vi "ADIS16470 Loop Custom.vi"(8 "error in":errorcluster) -> ()   [LabVIEW 2019]
uses:
  Typedef/ADIS16470 Hardware Configuration.ctl
  <vilib>/Rock Robotics/WPI/SPI/WPI_SPIMode.ctl
  <vilib>/Rock Robotics/SystemInterfaces/DIO/FPGA_DIOChannel.ctl
  <vilib>/Rock Robotics/SystemInterfaces/spilib/spi_bus.ctl
  Typedef/ADIS16470 Process.ctl
  Typedef/ADIS16470 Device Reference.ctl
  Typedef/ADIS16470 Data.ctl
  Typedef/ADIS16470 Status.ctl
  Typedef/ADIS16470 Command Type.ctl
  <vilib>/Rock Robotics/WPI/SPI/WPI_SPIDevRef.ctl
  <vilib>/Rock Robotics/WPI/Interrupt/WPI_InterruptRef.ctl
  <vilib>/Rock Robotics/SystemInterfaces/Interrupt/FPGA_InterruptIndex.ctl
  <vilib>/Rock Robotics/WPI/Encoder/WPI_EncoderDevRef.ctl
  <vilib>/Rock Robotics/SystemInterfaces/Encoder/FPGA_EncoderIdx.ctl
  <vilib>/Rock Robotics/SystemInterfaces/Counter/FPGA_CounterCtrSystemIndex.ctl
  <vilib>/Rock Robotics/WPI/Encoder/WPI_EncoderType.ctl
  <vilib>/Rock Robotics/SystemInterfaces/NetworkCommunication/NetComm_UsageReport_ResourceType.ctl
  Typedef/ADIS16470 Register.ctl
  <vilib>/Rock Robotics/WPI/Counter/WPI_CounterDigitalInputToDigitalSource.vi
  <vilib>/Rock Robotics/SystemInterfaces/CounterEncoderSourceConvertion/FPGA_CounterEncoderSourceConvertionLVSourceTypeToFPGAType.vi
  <vilib>/Rock Robotics/WPI/Interrupt/WPI_InterruptCache.vi
  <vilib>/Rock Robotics/SystemInterfaces/Interrupt/FPGA_InterruptWriteConfiguration.vi
  <vilib>/Rock Robotics/SystemInterfaces/Interrupt/FPGA_WaitOnInterrupt.vi
  <vilib>/Rock Robotics/WPI/Utilities/WPI_UtilitiesTimebaseConstants.vi
  <vilib>/Rock Robotics/SystemInterfaces/Interrupt/FPGA_InterruptReadTimestamp.vi
panel:
  in  "Sychronous Process VI":T1
  in  "Hardware Config":T2={"SPI Clock Rate (Hz)"=2000000.0, "IMU SPI Mode (3)"=enum."Mode 3 (Clk Idle High,Sample on Trailing)", "IMU Reset Pin"=enum."SPI Port CS2", "IMU SPI Bus"=enum."SPI On-Board, CS0", "IMU Data Ready Pin"=enum."SPI Port CS1"}
  out "Waveform Chart":dbl(graph)
  out "Offset Bias":i16[](array[numeric])
  out "xAngle":dbl
  out "yAngle":dbl
  out "Data":dbl[](array[numeric])
  out "Counter":u16
  # "x"
  # "y"
  # "z"
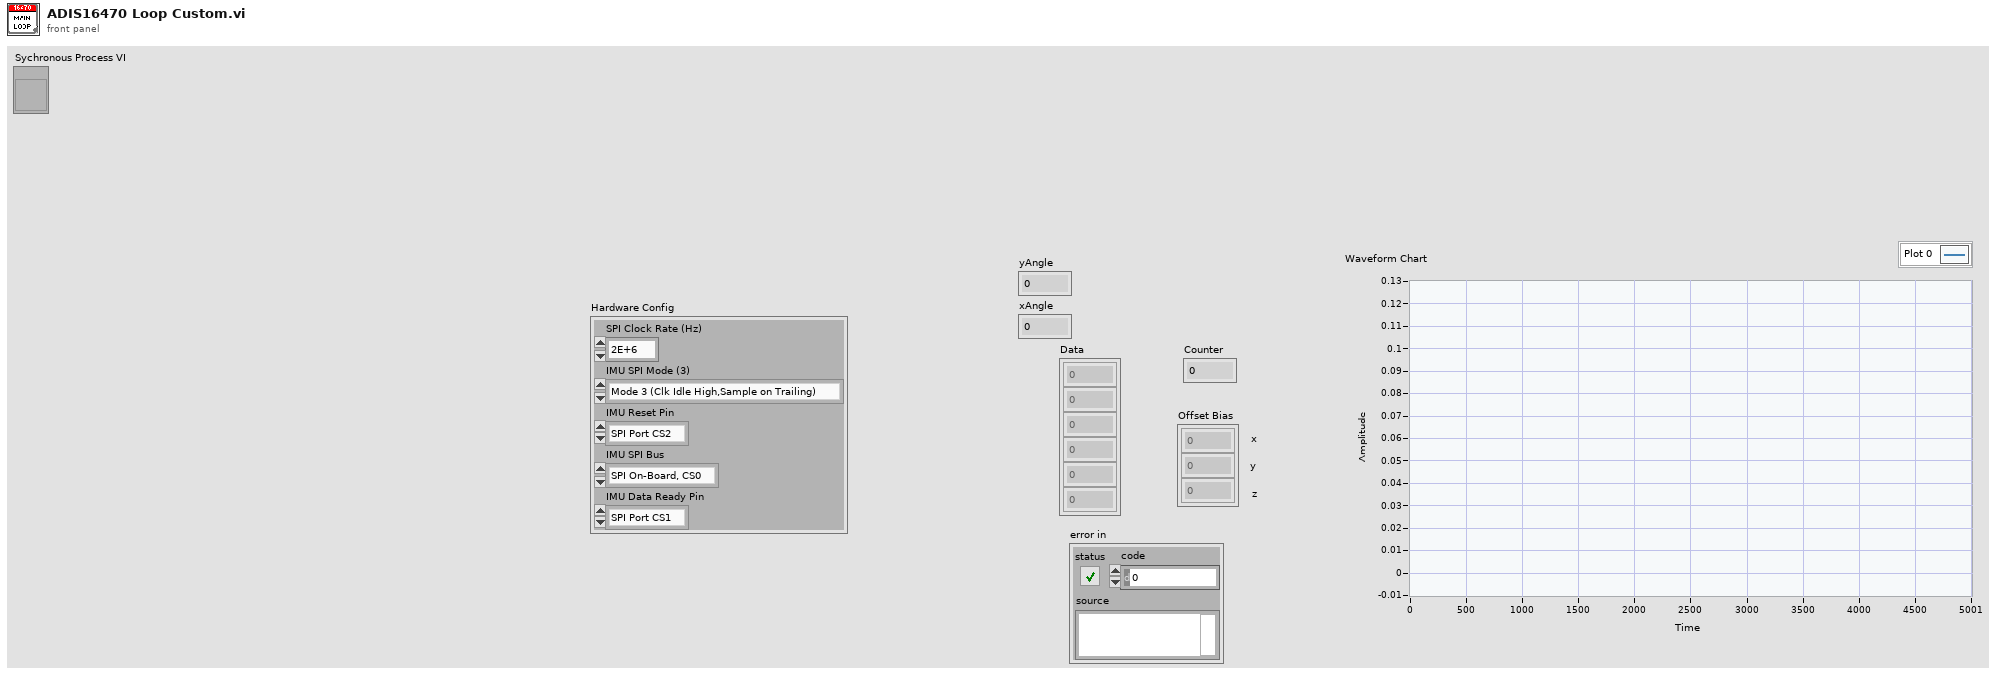
[diagram p1: front panel]
types:
  T1 = typedef "ADIS16470 Process.ctl" = refnum<vi>
  T2 = typedef "ADIS16470 Hardware Configuration.ctl" = cluster{"SPI Clock Rate (Hz)":dbl, "IMU SPI Mode (3)":T3, "IMU Reset Pin":T4, "IMU SPI Bus":T5, "IMU Data Ready Pin":T4}
  T3 = typedef "WPI_SPIMode.ctl" = enum16{"Mode 0 (Clk Idle Low,Sample on Leading)", "Mode 1 (Clk Idle Low,Sample on Trailing)", "Mode 2 (Clk Idle High,Sample on Leading)", "Mode 3 (Clk Idle High,Sample on Trailing)"}
  T4 = typedef "FPGA_DIOChannel.ctl" = enum8{"DIO 0", "DIO 1", "DIO 2", "DIO 3", "DIO 4", "DIO 5", "DIO 6", "DIO 7", "DIO 8", "DIO 9", "DIO MXP 0", "DIO MXP 1", "DIO MXP 2", "DIO MXP 3", "DIO MXP 4", "DIO MXP 5", "DIO MXP 6", "DIO MXP 7", "DIO MXP 8", "DIO MXP 9", "DIO MXP 10", "DIO MXP 11", "DIO MXP 12", "DIO MXP 13", "DIO MXP 14", "DIO MXP 15", "SPI Port CS1", "SPI Port CS2", "SPI Port CS3", "SPI Port MISO", "SPI Port MOSI", "Invalid"}
  T5 = typedef "spi_bus.ctl" = enum16{"SPI On-Board, CS0", "SPI On-Board, CS1", "SPI On-Board, CS2", "SPI On-Board, CS3", "SPI MXP", "Invalid"}
  T6 = typedef "NetComm_UsageReport_ResourceType.ctl" = enum8{"Controller", "Module", "Language", "CANPlugin", "Accelerometer", "ADXL345", "AnalogChannel", "AnalogTrigger", "AnalogTriggerOutput", "CANJaguar", "Compressor", "Counter", "Dashboard", "DigitalInput", "DigitalOutput", "DriverStationCIO", "DriverStationEIO", "DriverStationLCD", "Encoder", "GearTooth", "Gyro", "I2C", "Framework", "Jaguar", "Joystick", "Kinect", "KinectStick", "PIDController", "Preferences", "PWM", "Relay", "RobotDrive", "SerialPort", "Servo", "Solenoid", "SPI", "Task", "Ultrasonic", "Victor", "Button", "Command", "AxisCamera", "PCVideoServer", "SmartDashboard", "Talon", "HiTechnicColorSensor", "HiTechnicAccel", "HiTechnicCompass", "SRF08", "AnalogOutput", "Victor SP", "Talon SRX", "CAN Talon SRX", "ADXL362 Accel", "ADXRS450 Gyro", "Rev SPARK", "Mindsensors SD540", "Digital Filter", "ADIS16448", "PDP", "PCM", "PigeonIMU", "Nidec Brushless", "CTRE CANifier", "CTRE TalonFX", "CTRE Future 1", "CTRE Future 2", "CTRE Future 3", "CTRE Future 4", "CTRE Future 5", "CTRE Future 6", "Linear Filter", "Xbox Controller", "USB Camera", "NavX", "Pixy", "Pixy2", "ScanseSweep", "Shuffleboard", "CAN", "Digilent DMC60", "PWM Victor SPX", "Rev SPARK MAX PWM", "Rev SPARK MAX CAN", "ADIS16470", "PIDController2", "ProfiledPIDController", "Kinematics", "Odometry", "Units", "Trapezoid Profile", "DutyCycle", "Addressable LEDs", "Fusion Venom"}
  T7 = typedef "ADIS16470 Command Type.ctl" = enum16{"None", "Reset"}
  T8 = typedef "ADIS16470 Device Reference.ctl" = cluster{"DevStatus":errorcluster, "Hardware Config":T2, "End Calibration":refnum<notifier>, "Calibration Complete":refnum<notifier>, "Data FIFO":refnum<k33>, "Status FIFO":refnum<k33>, "Last Value Reference":refnum<data-value>, "Sychronous Process VI":T1, "Cmd FIFO":refnum<k33>}
  T9 = typedef "ADIS16470 Data.ctl" = cluster{"Yaw":dbl, "Timestamp":dbl, "Timestamp Delta":dbl, "Sample Count":u16}
  T10 = typedef "ADIS16470 Status.ctl" = cluster{"Calibrated?":bool}
  T11 = typedef "WPI_SPIDevRef.ctl" = cluster{"DevStatus":errorcluster, "Handle":i32, "SPI Bus":T5}
  T12 = typedef "WPI_InterruptRef.ctl" = cluster{"DevStatus":errorcluster, "InterruptIndex":T13}
  T13 = typedef "FPGA_InterruptIndex.ctl" = enum8{"0", "1", "2", "3", "4", "5", "6", "7", "Invalid"}
  T14 = typedef "WPI_EncoderDevRef.ctl" = cluster{"DevStatus":errorcluster, "EncoderIndex":T15, "CounterIndex":T16, "DistancePerCount":dbl, "Decoding Type":T17}
  T15 = typedef "FPGA_EncoderIdx.ctl" = enum8{"Enc 0", "Enc 1", "Enc 2", "Enc 3", "Enc 4", "Enc 5", "Enc 6", "Enc 7", "Invalid"}
  T16 = typedef "FPGA_CounterCtrSystemIndex.ctl" = enum8{"Ctr 0", "Ctr 1", "Ctr 2", "Ctr 3", "Ctr 4", "Ctr 5", "Ctr 6", "Ctr 7", "Invalid"}
  T17 = typedef "WPI_EncoderType.ctl" = enum16{"1x", "2x", "4x"}
  T18 = cluster{"ADIS16470DevRef":T8, "SPIDevRef":T11, "InterruptRef":T12, "Sensor to Robot Rotation":dbl[][], "Yaw":dbl, "Data Counter":u16, "First Run":bool, "TimeStamp Prev":dbl, "Time Delta":dbl, "Encoder Right":T14, "Encoder Left":T14, "Encoder Data":cluster{"Left Distance":dbl, "Right Distance":dbl}}
  T19 = typedef "WPI_DigitalInputDevRef.ctl" = cluster{"DevStatus":errorcluster, "DIO Channel":T4}
  T20 = typedef "FPGA_CounterEncoderSourceConvertionLVSourceType.ctl" = cluster{"DevStatus":errorcluster, "AnalogTriggerMode?":bool, "DigitalMode":cluster{"DIO Channel":T21}, "AnalogTriggerMode":cluster{"AnalogTriggerIndex":T22, "OutputType":T23}}
  T21 = typedef "FPGA_DIODigitalSourceChannel.ctl" = enum8{"DIO 0", "DIO 1", "DIO 2", "DIO 3", "DIO 4", "DIO 5", "DIO 6", "DIO 7", "DIO 8", "DIO 9", "DIO MXP 0", "DIO MXP 1", "DIO MXP 2", "DIO MXP 3", "DIO MXP 4", "DIO MXP 5", "DIO MXP 6", "DIO MXP 7", "DIO MXP 8", "DIO MXP 9", "DIO MXP 10", "DIO MXP 11", "DIO MXP 12", "DIO MXP 13", "DIO MXP 14", "DIO MXP 15", "SPI Port CS1", "SPI Port CS2", "SPI Port CS3", "SPI Port MISO", "SPI Port MOSI", "Disabled"}
  T22 = typedef "FPGA_AnalogTriggerIndex.ctl" = enum8{"Trig 0", "Trig 1", "Trig 2", "Trig 3", "Trig 4", "Trig 5", "Trig 6", "Trig 7", "Invalid"}
  T23 = typedef "FPGA_AnalogTriggerOutType.ctl" = enum16{"InWindow", "TriggerState", "Rising", "Falling"}
  T24 = typedef "ADIS16470 Register.ctl" = u8
  T25 = typedef "WPI_DigitalOutputDevRef.ctl" = cluster{"DIO Channel":T4, "DevStatus":errorcluster}
  T26 = cluster{"Left Distance":dbl, "Right Distance":dbl}
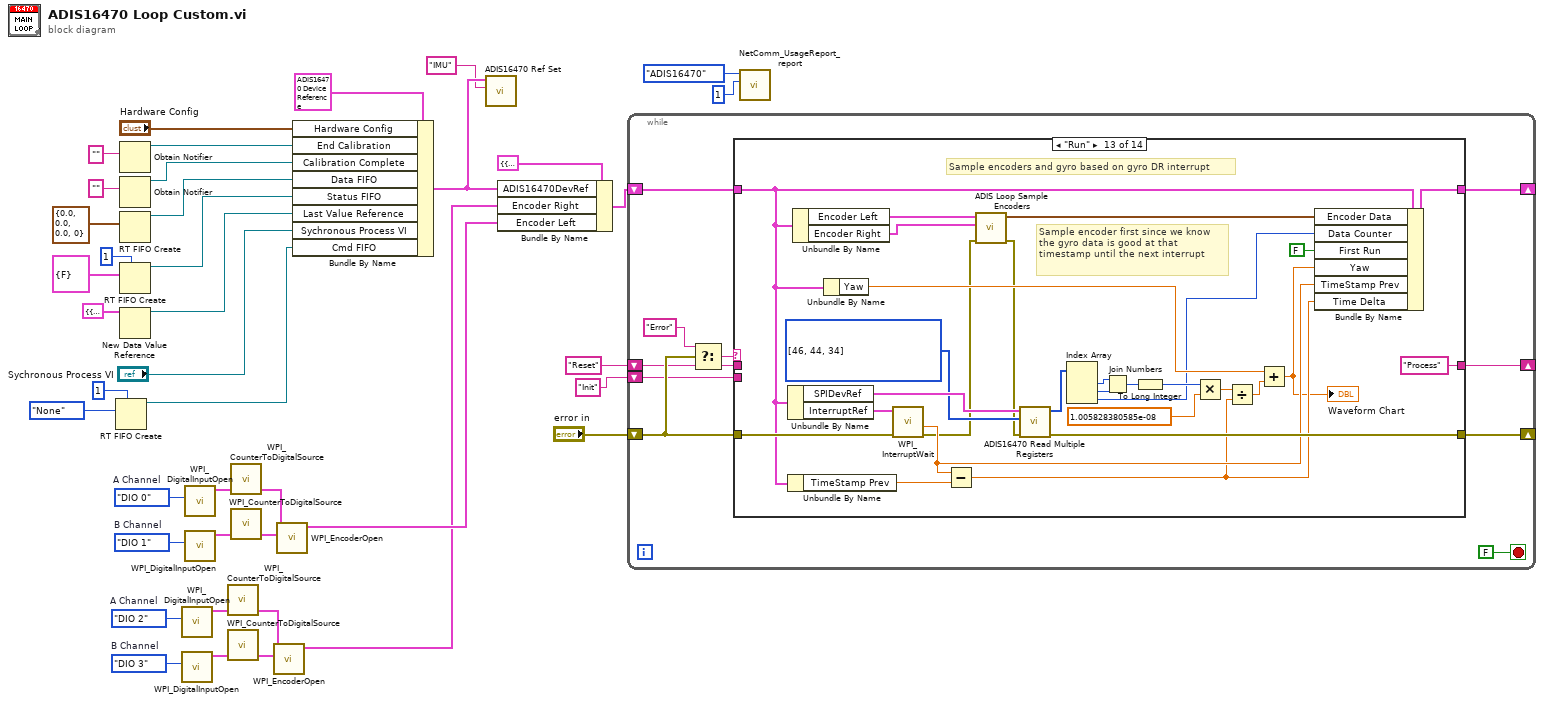
[diagram p0: block diagram]
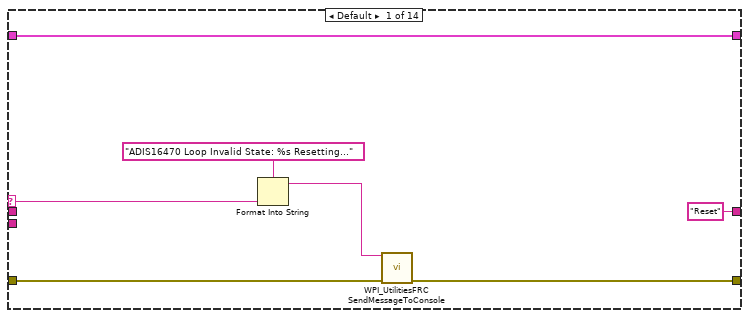
[diagram p2: hidden frame]
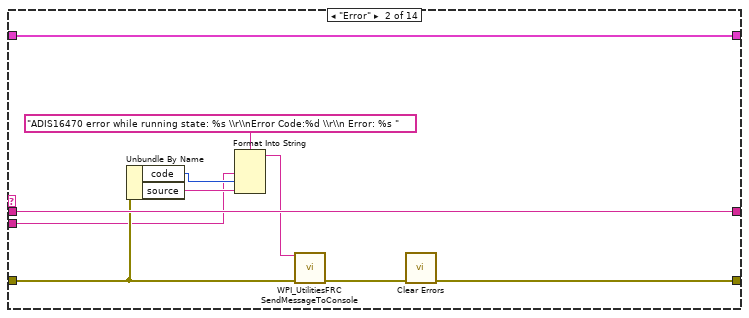
[diagram p3: hidden frame]
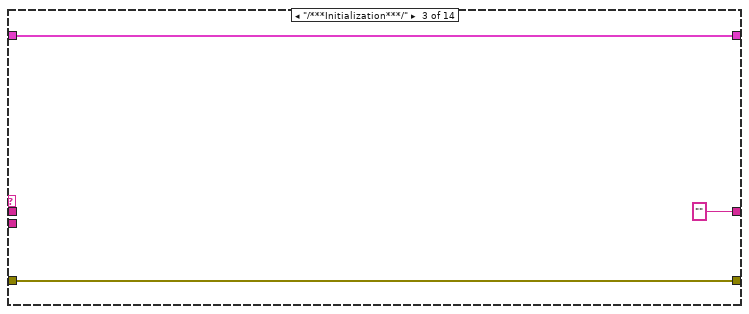
[diagram p4: hidden frame]
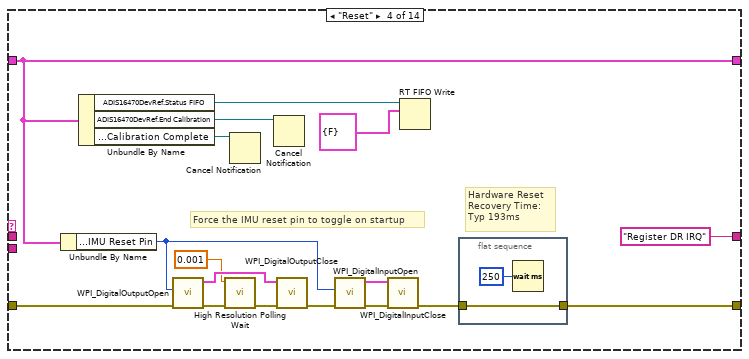
[diagram p5: hidden frame]
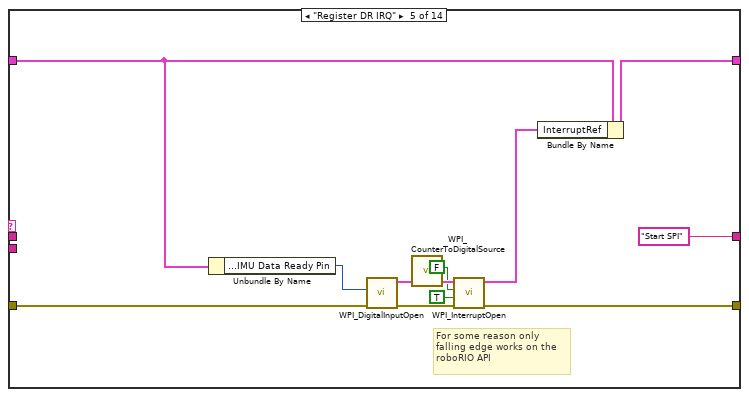
[diagram p6: hidden frame]
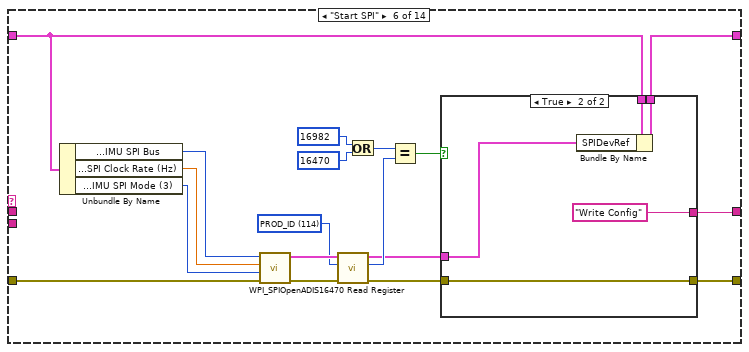
[diagram p7: hidden frame]
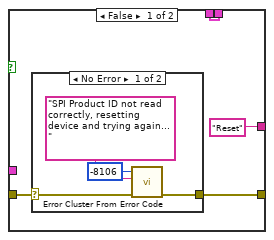
[diagram p8: hidden frame]
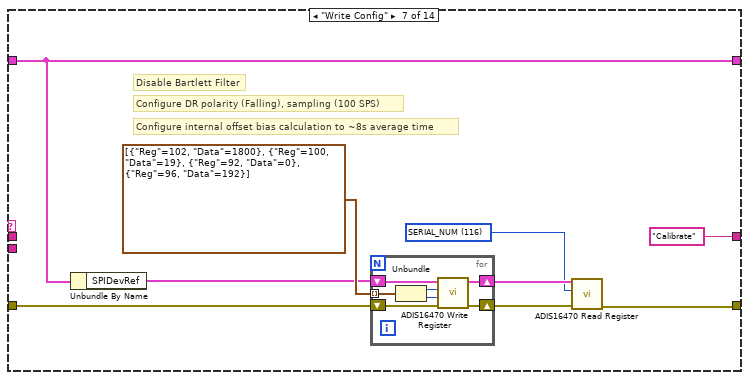
[diagram p10: hidden frame]
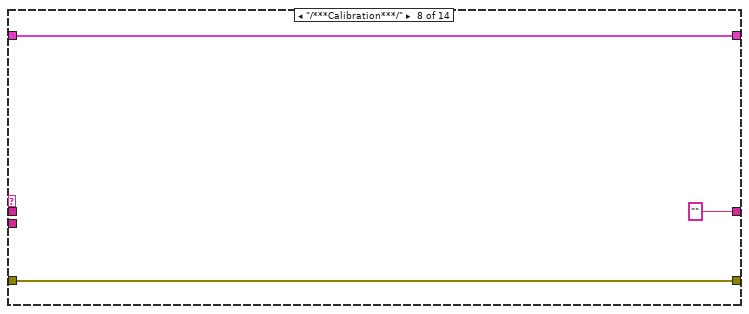
[diagram p11: hidden frame]
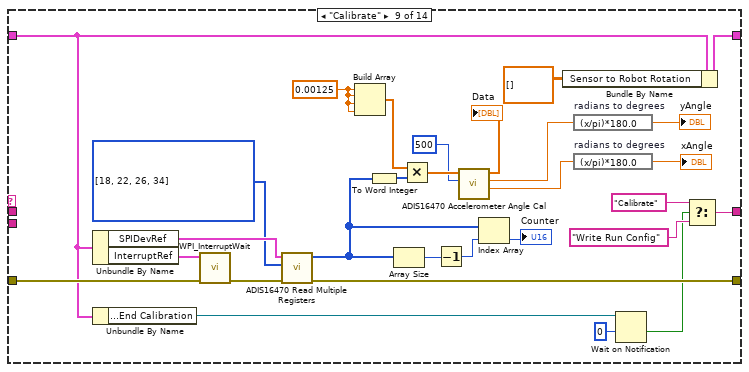
[diagram p12: hidden frame]
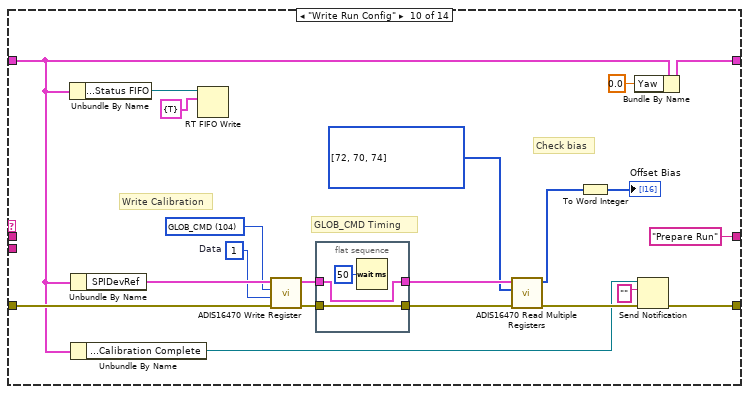
[diagram p13: hidden frame]
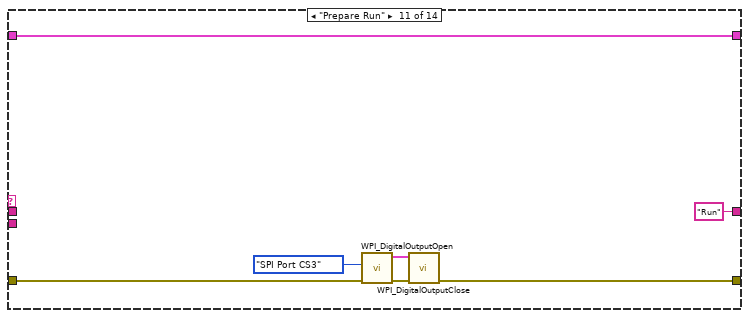
[diagram p14: hidden frame]
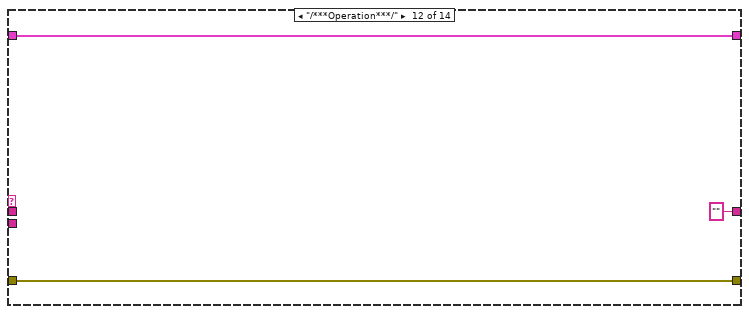
[diagram p15: hidden frame]
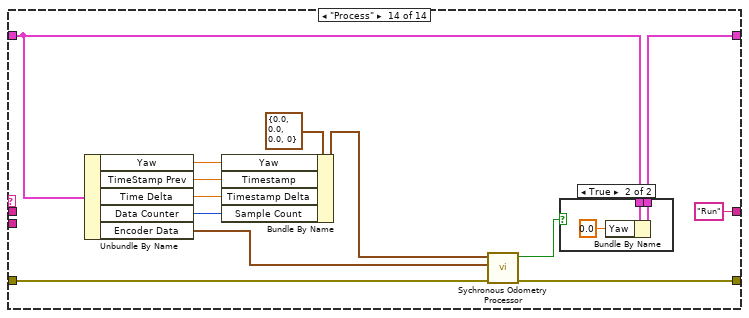
[diagram p16: hidden frame]
diagram:
  w7 = FPGA_DIOChannel."DIO 3"  # B Channel
  w6 = FPGA_DIOChannel."DIO 2"  # A Channel
  w14 = FPGA_DIOChannel."DIO 1"  # B Channel
  w13 = FPGA_DIOChannel."DIO 0"  # A Channel
  n1 = RT FIFO Create(1:ADIS16470_Command_Type."None", 4:u32 1 ("size (10)")) -> (8:w19:refnum<k33>)  [unwired: 6 in, 2 out]
  n2 = Obtain Notifier(notification data type="") -> (notifier out=w32:refnum<notifier>)  [unwired: 3 in, 2 out]
  n3 = Obtain Notifier(notification data type="") -> (notifier out=w33:refnum<notifier>)  [unwired: 3 in, 2 out]
  n4 = RT FIFO Create(1:T9 {"Yaw"=0.0, "Timestamp"=0.0, "Timestamp Delta"=0.0, "Sample Count"=0}) -> (8:w26:refnum<k33>)  [unwired: 7 in, 2 out]
  n5 = RT FIFO Create(1:T10 {"Calibrated?"=FALSE}, 4:u32 1 ("size (10)")) -> (8:w25:refnum<k33>)  [unwired: 6 in, 2 out]
  n6 = New Data Value Reference(data value=cluster{T9, T10} {{"Yaw"=0.0, "Timestamp"=0.0, "Timestamp Delta"=0.0, "Sample Count"=0}, {"Calibrated?"=FALSE}} ("output cluster")) -> (data value reference=w23:refnum<data-value>)  [unwired: 1 in, 1 out]
  n7 = call <vilib>:"WPI_DigitalInputOpen.vi"("DIO Channel"=w6) -> ("DigitalInputDevRef"=w3:T19)  [unwired: 1 in, 9 out]
  n8 = call <vilib>:"WPI_DigitalInputOpen.vi"("DIO Channel"=w7) -> ("DigitalInputDevRef"=w4:T19)  [unwired: 1 in, 9 out]
  n9 = call <vilib>:"WPI_DigitalInputOpen.vi"("DIO Channel"=w13) -> ("DigitalInputDevRef"=w10:T19)  [unwired: 1 in, 9 out]
  n10 = call <vilib>:"WPI_DigitalInputOpen.vi"("DIO Channel"=w14) -> ("DigitalInputDevRef"=w11:T19)  [unwired: 1 in, 9 out]
  n11 = call-poly <vilib>:"WPI_CounterToDigitalSource.vi"("DigitalInputDevRef"=w3) -> ("Digital Source"=w2:T20)  [unwired: 6 out]
  n12 = call-poly <vilib>:"WPI_CounterToDigitalSource.vi"("DigitalInputDevRef"=w4) -> ("Digital Source"=w5:T20)  [unwired: 6 out]
  n13 = call-poly <vilib>:"WPI_CounterToDigitalSource.vi"("DigitalInputDevRef"=w10) -> ("Digital Source"=w9:T20)  [unwired: 6 out]
  n14 = call-poly <vilib>:"WPI_CounterToDigitalSource.vi"("DigitalInputDevRef"=w11) -> ("Digital Source"=w12:T20)  [unwired: 6 out]
  n15 = call <vilib>:"WPI_EncoderOpen.vi"("BSource"=w5, "ASource"=w2) -> ("EncoderDevRef"=w1:T14)  [unwired: 6 in, 3 out]
  n16 = call <vilib>:"WPI_EncoderOpen.vi"("BSource"=w12, "ASource"=w9) -> ("EncoderDevRef"=w8:T14)  [unwired: 6 in, 3 out]
  n17 = Bundle By Name(cluster=T8 {"DevStatus"={"status"=FALSE, "code"=0, "source"=""}, "Hardware Config"={"SPI Clock Rate (Hz)"=1000000.0, "IMU SPI Mode (3)"=enum."Mode 3 (Clk Idle High,Sample on Trailing)", "IMU Reset Pin"=enum."SPI Port CS2", "IMU SPI Bus"=enum."SPI On-Board, CS0", "IMU Data Ready Pin"=enum."SPI Port CS1"}, "End Calibration"=refnum, "Calibration Complete"=refnum, "Data FIFO"=refnum, "Status FIFO"=refnum, "Last Value Reference"=refnum, "Sychronous Process VI"=refnum, "Cmd FIFO"=refnum} ("ADIS16470DevRef"), "Hardware Config"="Hardware Config", "End Calibration"=w32, "Calibration Complete"=w33, "Data FIFO"=w26, "Status FIFO"=w25, "Last Value Reference"=w23, "Sychronous Process VI"="Sychronous Process VI", "Cmd FIFO"=w19) -> (w16:T8)
  n18 = call "ADIS16470 Ref Set.vi"("refnum name"="IMU", "ADIS16470DevRef in"=w16) -> ()  [unwired: 8 in, 2 out]
  n19 = Bundle By Name(cluster=T18 {"ADIS16470DevRef"={"DevStatus"={"status"=FALSE, "code"=0, "source"=""}, "Hardware Config"={"SPI Clock Rate (Hz)"=1000000.0, "IMU SPI Mode (3)"=enum."Mode 3 (Clk Idle High,Sample on Trailing)", "IMU Reset Pin"=enum."SPI Port CS2", "IMU SPI Bus"=enum."SPI On-Board, CS0", "IMU Data Ready Pin"=enum."SPI Port CS1"}, "End Calibration"=refnum, "Calibration Complete"=refnum, "Data FIFO"=refnum, "Status FIFO"=refnum, "Last Value Reference"=refnum, "Sychronous Process VI"=refnum, "Cmd FIFO"=refnum}, "SPIDevRef"={"DevStatus"={"status"=FALSE, "code"=0, "source"=""}, "Handle"=0, "SPI Bus"=enum."SPI On-Board, CS0"}, "InterruptRef"={"DevStatus"={"status"=FALSE, "code"=0, "source"=""}, "InterruptIndex"=enum."Invalid"}, "Sensor to Robot Rotation"=[[0.0, 0.0, 0.0], [0.0, 0.0, 0.0], [0.0, 0.0, 0.0]], "Yaw"=0.0, "Data Counter"=0, "First Run"=FALSE, "TimeStamp Prev"=0.0, "Time Delta"=0.0, "Encoder Right"={"DevStatus"={"status"=FALSE, "code"=0, "source"=""}, "EncoderIndex"=enum."Invalid", "CounterIndex"=enum."Invalid", "DistancePerCount"=1.0, "Decoding Type"=enum."4x"}, "Encoder Left"={"DevStatus"={"status"=FALSE, "code"=0, "source"=""}, "EncoderIndex"=enum."Invalid", "CounterIndex"=enum."Invalid", "DistancePerCount"=1.0, "Decoding Type"=enum."4x"}, "Encoder Data"={"Left Distance"=0.0, "Right Distance"=0.0}}, "ADIS16470DevRef"=w16, "Encoder Right"=w1, "Encoder Left"=w8) -> (w38:T18)
  n20 = while {
    shift-right: [w46] -> _
    shift-left: "Reset" -> [w43]
    shift-right: [w48] -> _
    shift-left: w38 -> [w49]
    shift-right: [w47] -> _
    shift-left: "error in" -> [w45]
    shift-left: "Init" -> [w41]
    stop <- FALSE stop-if-true
    n21 = Select(t="Error", s=w45, f=w43) -> (s? t:f=w44:string)
    n22 = case shown="\"Run\"" w44 {
      selector: w44 -> [w56 _ _ _ _ _ _ _ _ _ _ _ _ _]
      tunnel: w49 -> [w57 w67 w70 w75 w93 w109 w141 w152 w165 w186 w212 w215 w222 w255]
      tunnel: [w57 w67 w70 w75 w100 w110 w141 w152 w167 w193 w212 w215 w233 w245] -> w48
      tunnel: w45 -> [w55 w63 w69 w82 w96 w116 w138 w151 w180 w200 w208 w214 w241 w249]
      tunnel: [w54 w64 w69 w77 w99 w108 w135 w151 w177 w188 w207 w214 w239 w248] -> w47
      tunnel: ["Reset" w66 "" "Register DR IRQ" "Start SPI" w111 "Calibrate" "" w164 "Prepare Run" "Run" "" "Process" "Run"] -> w46
      tunnel: w43 -> [_ w66 _ _ _ _ _ _ _ _ _ _ _ _]
      tunnel: w41 -> [_ w58 _ _ _ _ _ _ _ _ _ _ _ _]
      frame Default {
        n23 = Format Into String(format string="ADIS16470 Loop Invalid State: %s Resetting...", w56) -> (resulting string=w53:string)  [unwired: 2 in, 1 out]
        n24 = call <vilib>:"WPI_UtilitiesFRC SendMessageToConsole.vi"("Message"=w53, "error in (no error)"=w55) -> ("error out"=w54:errorcluster)  [unwired: 13 in]
      }
      frame "Error" {
        n25 = Unbundle By Name(w63) -> ("code"=w60:i32, "source"=w59:string)
        n26 = Format Into String(format string="ADIS16470 error while running state: %s \\r\\nError Code:%d \\r\\n Error: %s ", w58, w60, w59) -> (resulting string=w62:string)  [unwired: 2 in, 1 out]
        n27 = call <vilib>:"WPI_UtilitiesFRC SendMessageToConsole.vi"("Message"=w62, "error in (no error)"=w63) -> ("error out"=w65:errorcluster)  [unwired: 13 in]
        n28 = call <vilib>:"Clear Errors.vi"("error in (no error)"=w65) -> ("error out"=w64:errorcluster)  [unwired: 5 in, 1 out]
      }
      frame "/***Initialization***/" {
      }
      frame "Reset" {
        # "Hardware Reset Recovery Time: Typ 193ms"
        # "Force the IMU reset pin to toggle on startup"
        n29 = Unbundle By Name(w75) -> ("ADIS16470DevRef.Hardware Config.IMU Reset Pin"=w83:T4)
        n30 = Unbundle By Name(w75) -> ("ADIS16470DevRef.Status FIFO"=w72:refnum<k33>, "ADIS16470DevRef.End Calibration"=w73:refnum<notifier>, "ADIS16470DevRef.Calibration Complete"=w74:refnum<notifier>)
        n31 = call <vilib>:"WPI_DigitalOutputOpen.vi"("error in (no error)"=w82, "DIO Channel"=w83) -> ("error out"=w80:errorcluster, "DigitalOutputDevRef"=w84:T25)  [unwired: 8 in]
        n32 = call <vilib>:"High Resolution Polling Wait.vi"("error in (no error)"=w80, "seconds to wait"=0.001) -> ("error out"=w79:errorcluster)  [unwired: 9 in]
        n33 = Cancel Notification(0:w74) -> ()  [unwired: 1 in, 3 out]
        n34 = Cancel Notification(0:w73) -> ()  [unwired: 1 in, 3 out]
        n35 = call <vilib>:"WPI_DigitalOutputClose.vi"("error in (no error)"=w79, "DigitalOutputDevRef"=w84) -> ("error out"=w87:errorcluster)  [unwired: 9 in]
        n36 = call <vilib>:"WPI_DigitalInputOpen.vi"("error in (no error)"=w87, "DIO Channel"=w83) -> ("error out"=w86:errorcluster, "DigitalInputDevRef"=w85:T19)  [unwired: 8 in]
        n37 = call <vilib>:"WPI_DigitalInputClose.vi"("error in (no error)"=w86, "DigitalInputDevRef"=w85) -> ("error out"=w76:errorcluster)  [unwired: 9 in]
        n38 = RT FIFO Write(0:w72, 1:T10 {"Calibrated?"=FALSE} ("element")) -> ()  [unwired: 3 in, 4 out]
        n39 = flat-sequence {
          tunnel: [w89] -> w77
          tunnel: w76 -> [w89]
          frame #0 {
            n40 = Wait (ms)(milliseconds to wait=u32 250) -> ()  [unwired: 1 out]
          }
        }
      }
      frame "Register DR IRQ" {
        # "For some reason only\nfalling edge works on the\nroboRIO API"
        n41 = Unbundle By Name(w93) -> ("ADIS16470DevRef.Hardware Config.IMU Data Ready Pin"=w92:T4)
        n42 = call <vilib>:"WPI_DigitalInputOpen.vi"("error in (no error)"=w96, "DIO Channel"=w92) -> ("error out"=w95:errorcluster, "DigitalInputDevRef"=w94:T19)  [unwired: 8 in]
        n43 = call-poly <vilib>:"WPI_CounterToDigitalSource.vi"("DigitalInputDevRef"=w94) -> ("Digital Source"=w97:T20)  [unwired: 6 in]
        n44 = call <vilib>:"WPI_InterruptOpen.vi"("error in (no error)"=w95, "Falling Edge"=TRUE, "Rising Edge"=FALSE, "Source"=w97) -> ("error out"=w99:errorcluster, "InterruptRef"=w98:T12)  [unwired: 6 in]
        n45 = Bundle By Name(cluster=w93, "InterruptRef"=w98) -> (w100:T18)
      }
      frame "Start SPI" {
        w103 = T24 114 items=["Reserved1"=0, "DIAG_STAT"=2, "X_GYRO_LOW"=4, "X_GYRO_OUT"=6, "Y_GYRO_LOW"=8, "Y_GYRO_OUT"=10, "Z_GYRO_LOW"=12, "Z_GYRO_OUT"=14, "X_ACCL_LOW"=16, "X_ACCL_OUT"=18, "Y_ACCL_LOW"=20, "Y_ACCL_OUT"=22, "Z_ACCL_LOW"=24, "Z_ACCL_OUT"=26, "TEMP_OUT"=28, "TIME_STAMP"=30, "Reseved2"=32, "DATA_CNTR"=34, "X_DELTANG_LOW"=36, "X_DELTANG_OUT"=38, "Y_DELTANG_LOW"=40, "Y_DELTANG_OUT"=42, "Z_DELTANG_LOW"=44, "Z_DELTANG_OUT"=46, "X_DELTVEL_LOW"=48, "X_DELTVEL_OUT"=50, "Y_DELTVEL_LOW"=52, "Y_DELTVEL_OUT"=54, "Z_DELTVEL_LOW"=56, "Z_DELTVEL_OUT"=58, "Reserved3"=60, "Reserved4"=62, "XG_BIAS_LOW"=64, "XG_BIAS_HIGH"=66, "YG_BIAS_LOW"=68, "YG_BIAS_OUT"=70, "ZG_BIAS_LOW"=72, "ZG_BIAS_OUT"=74, "XA_BIAS_LOW"=76, "XA_BIAS_HIGH"=78, "YA_BIAS_LOW"=80, "YA_BIAS_OUT"=82, "ZA_BIAS_LOW"=84, "ZA_BIAS_OUT"=86, "Reserved5"=88, "Reserved6"=90, "FILT_CTRL"=92, "Reserved5"=94, "MSC_CTRL"=96, "UP_SCALE"=98, "DEC_RATE"=100, "NULL_CNFG"=102, "GLOB_CMD"=104, "Reserved6"=106, "FIRM_REV"=108, "FIRM_DM"=110, "FIRM_Y"=112, "PROD_ID"=114, "SERIAL_NUM"=116, "USER_SCR1"=118, "USER_SCR2"=120, "USER_SCR3"=122, "FLSHCNT_LOW"=124, "FLSHCNT_HIGH"=126] ("ADIS16448 Register")
        n46 = Unbundle By Name(w109) -> ("ADIS16470DevRef.Hardware Config.IMU SPI Bus"=w112:T5, "ADIS16470DevRef.Hardware Config.SPI Clock Rate (Hz)"=w113:dbl, "ADIS16470DevRef.Hardware Config.IMU SPI Mode (3)"=w114:T3)
        n47 = call <vilib>:"WPI_SPIOpen.vi"("error in"=w116, "Mode (3)"=w114, "Clock Rate (Hz)"=w113, "SPI Bus"=w112) -> ("error out"=w105:errorcluster, "SPIDevRef"=w104:T11)  [unwired: 6 in]
        n48 = call "ADIS16470 Read Register.vi"("error in (no error)"=w105, "ADIS16470 Register"=w103, "SPIDevRef in"=w104) -> ("error out"=w106:errorcluster, "Register Value"=w107:u16, "SPIDevRef out"=w102:T11)  [unwired: 6 in]
        n49 = Or(x=u16 16982 ("y"), y=u16 16470) -> (x .or. y?=w117:u16)
        n50 = Equal?(x=w117, y=w107) -> (x = y?=w115:bool)
        n51 = case shown="True" w115 {
          tunnel: ["Reset" "Write Config"] -> w111
          tunnel: w109 -> [w122 w132]
          tunnel: [w122 w131] -> w110
          tunnel: [w121 w129] -> w108
          tunnel: w106 -> [w120 w129]
          tunnel: w102 -> [_ w130]
          frame False {
            n52 = case shown="No Error" w120 {
              selector: w120 -> [w126 w128]
              tunnel: [w127 w128] -> w121
              frame No Error {
                n53 = call <vilib>:"Error Cluster From Error Code.vi"("error in (no error)"=w126, "error message (\"\")"="SPI Product ID not read correctly, resetting device and trying again..." ("error message (\"\")"), "error code (0)"=-8106) -> ("error out"=w127:errorcluster)  [unwired: 6 in]
              }
              frame Error {
              }
            }
          }
          frame True {
            n54 = Bundle By Name(cluster=w132, "SPIDevRef"=w130) -> (w131:T18)
          }
        }
      }
      frame "Write Config" {
        w134 = T24 116 items=["Reserved1"=0, "DIAG_STAT"=2, "X_GYRO_LOW"=4, "X_GYRO_OUT"=6, "Y_GYRO_LOW"=8, "Y_GYRO_OUT"=10, "Z_GYRO_LOW"=12, "Z_GYRO_OUT"=14, "X_ACCL_LOW"=16, "X_ACCL_OUT"=18, "Y_ACCL_LOW"=20, "Y_ACCL_OUT"=22, "Z_ACCL_LOW"=24, "Z_ACCL_OUT"=26, "TEMP_OUT"=28, "TIME_STAMP"=30, "Reseved2"=32, "DATA_CNTR"=34, "X_DELTANG_LOW"=36, "X_DELTANG_OUT"=38, "Y_DELTANG_LOW"=40, "Y_DELTANG_OUT"=42, "Z_DELTANG_LOW"=44, "Z_DELTANG_OUT"=46, "X_DELTVEL_LOW"=48, "X_DELTVEL_OUT"=50, "Y_DELTVEL_LOW"=52, "Y_DELTVEL_OUT"=54, "Z_DELTVEL_LOW"=56, "Z_DELTVEL_OUT"=58, "Reserved3"=60, "Reserved4"=62, "XG_BIAS_LOW"=64, "XG_BIAS_HIGH"=66, "YG_BIAS_LOW"=68, "YG_BIAS_OUT"=70, "ZG_BIAS_LOW"=72, "ZG_BIAS_OUT"=74, "XA_BIAS_LOW"=76, "XA_BIAS_HIGH"=78, "YA_BIAS_LOW"=80, "YA_BIAS_OUT"=82, "ZA_BIAS_LOW"=84, "ZA_BIAS_OUT"=86, "Reserved5"=88, "Reserved6"=90, "FILT_CTRL"=92, "Reserved5"=94, "MSC_CTRL"=96, "UP_SCALE"=98, "DEC_RATE"=100, "NULL_CNFG"=102, "GLOB_CMD"=104, "Reserved6"=106, "FIRM_REV"=108, "FIRM_DM"=110, "FIRM_Y"=112, "PROD_ID"=114, "SERIAL_NUM"=116, "USER_SCR1"=118, "USER_SCR2"=120, "USER_SCR3"=122, "FLSHCNT_LOW"=124, "FLSHCNT_HIGH"=126] ("ADIS16448 Register")
        # "Configure internal offset bias calculation to ~8s average time"
        # "Configure DR polarity (Falling), sampling (100 SPS)"
        # "Disable Bartlett Filter"
        n55 = Unbundle By Name(w141) -> ("SPIDevRef"=w139:T11)
        n56 = for {
          tunnel: cluster{"Reg":T24, "Data":u16}[] [{"Reg"=102, "Data"=1800}, {"Reg"=100, "Data"=19}, {"Reg"=92, "Data"=0}, {"Reg"=96, "Data"=192}] -> [w149] mode=indexing
          shift-right: [w145] -> w136
          shift-left: w138 -> [w144]
          shift-right: [w143] -> w137
          shift-left: w139 -> [w146]
          n57 = Unbundle(w149) -> ("Reg"=w148:T24, "Data"=w147:u16)
          n58 = call "ADIS16470 Write Register.vi"("error in (no error)"=w144, "Data"=w147, "Register"=w148, "SPIDevRef in"=w146) -> ("error out"=w145:errorcluster, "SPIDevRef out"=w143:T11)  [unwired: 6 in]
        }
        n59 = call "ADIS16470 Read Register.vi"("error in (no error)"=w136, "ADIS16470 Register"=w134, "SPIDevRef in"=w137) -> ("error out"=w135:errorcluster)  [unwired: 6 in, 2 out]
      }
      frame "/***Calibration***/" {
      }
      frame "Calibrate" {
        w171 = 0.00125
        w172 = T24[] [18, 22, 26, 34] items=["Reserved1"=0, "DIAG_STAT"=2, "X_GYRO_LOW"=4, "X_GYRO_OUT"=6, "Y_GYRO_LOW"=8, "Y_GYRO_OUT"=10, "Z_GYRO_LOW"=12, "Z_GYRO_OUT"=14, "X_ACCL_LOW"=16, "X_ACCL_OUT"=18, "Y_ACCL_LOW"=20, "Y_ACCL_OUT"=22, "Z_ACCL_LOW"=24, "Z_ACCL_OUT"=26, "TEMP_OUT"=28, "TIME_STAMP"=30, "Reseved2"=32, "DATA_CNTR"=34, "X_DELTANG_LOW"=36, "X_DELTANG_OUT"=38, "Y_DELTANG_LOW"=40, "Y_DELTANG_OUT"=42, "Z_DELTANG_LOW"=44, "Z_DELTANG_OUT"=46, "X_DELTVEL_LOW"=48, "X_DELTVEL_OUT"=50, "Y_DELTVEL_LOW"=52, "Y_DELTVEL_OUT"=54, "Z_DELTVEL_LOW"=56, "Z_DELTVEL_OUT"=58, "Reserved3"=60, "Reserved4"=62, "XG_BIAS_LOW"=64, "XG_BIAS_HIGH"=66, "YG_BIAS_LOW"=68, "YG_BIAS_OUT"=70, "ZG_BIAS_LOW"=72, "ZG_BIAS_OUT"=74, "XA_BIAS_LOW"=76, "XA_BIAS_HIGH"=78, "YA_BIAS_LOW"=80, "YA_BIAS_OUT"=82, "ZA_BIAS_LOW"=84, "ZA_BIAS_OUT"=86, "Reserved5"=88, "Reserved6"=90, "FILT_CTRL"=92, "Reserved5"=94, "MSC_CTRL"=96, "UP_SCALE"=98, "DEC_RATE"=100] ("Registers")
        n60 = Unbundle By Name(w165) -> ("SPIDevRef"=w178:T11, "InterruptRef"=w181:T12)
        n61 = Unbundle By Name(w165) -> ("ADIS16470DevRef.End Calibration"=w155:refnum<notifier>)
        n62 = call <vilib>:"WPI_InterruptWait.vi"("error in (no error)"=w180, "InterruptRef"=w181) -> ("error out"=w179:errorcluster)  [unwired: 5 in, 4 out]
        n63 = call "ADIS16470 Read Multiple Registers.vi"("error in (no error)"=w179, "Registers"=w172, "SPIDevRef"=w178) -> ("error out"=w177:errorcluster, "Values"=w160:u16[])  [unwired: 7 in]
        n64 = Build Array(w171, w171, w171, w171) -> (w176:dbl[])
        n65 = To Word Integer(number=w160) -> (16bit integer=w161:i16[])
        n66 = Array Size(array=w160) -> (size(s)=w175:i32)
        n67 = Multiply(x=w176, y=w161) -> (x*y=w170:dbl[])
        n68 = Decrement(x=w175) -> (x-1=w174:i32)
        n69 = call "ADIS16470 Accelerometer Angle Cal.vi"("average samples"=500, "Raw Accel In"=w170) -> ("xAngle"=w158:dbl, "yAngle"=w157:dbl, "Average Accel Out"=→"Data":dbl[])  [unwired: 7 in]
        n70 = Index Array(array=w160, index=w174) -> (element=→"Counter":u16)
        n71 = Bundle By Name(cluster=w165, "Sensor to Robot Rotation"=dbl[][] []) -> (w167:T18)
        n72 = expression code="(x/pi)*180.0" "radians to degrees"(w157) -> (→"yAngle":dbl)
        n73 = expression code="(x/pi)*180.0" "radians to degrees"(w158) -> (→"xAngle":dbl)
        n74 = Wait on Notification(notifier=w155, timeout in ms (-1)=0) -> (timed out?=w153:bool)  [unwired: 2 in, 3 out]
        n75 = Select(t="Calibrate", s=w153, f="Write Run Config") -> (s? t:f=w164:string)
      }
      frame "Write Run Config" {
        w183 = T24 104 items=["Reserved1"=0, "DIAG_STAT"=2, "X_GYRO_LOW"=4, "X_GYRO_OUT"=6, "Y_GYRO_LOW"=8, "Y_GYRO_OUT"=10, "Z_GYRO_LOW"=12, "Z_GYRO_OUT"=14, "X_ACCL_LOW"=16, "X_ACCL_OUT"=18, "Y_ACCL_LOW"=20, "Y_ACCL_OUT"=22, "Z_ACCL_LOW"=24, "Z_ACCL_OUT"=26, "TEMP_OUT"=28, "TIME_STAMP"=30, "Reseved2"=32, "DATA_CNTR"=34, "X_DELTANG_LOW"=36, "X_DELTANG_OUT"=38, "Y_DELTANG_LOW"=40, "Y_DELTANG_OUT"=42, "Z_DELTANG_LOW"=44, "Z_DELTANG_OUT"=46, "X_DELTVEL_LOW"=48, "X_DELTVEL_OUT"=50, "Y_DELTVEL_LOW"=52, "Y_DELTVEL_OUT"=54, "Z_DELTVEL_LOW"=56, "Z_DELTVEL_OUT"=58, "Reserved3"=60, "Reserved4"=62, "XG_BIAS_LOW"=64, "XG_BIAS_HIGH"=66, "YG_BIAS_LOW"=68, "YG_BIAS_OUT"=70, "ZG_BIAS_LOW"=72, "ZG_BIAS_OUT"=74, "XA_BIAS_LOW"=76, "XA_BIAS_HIGH"=78, "YA_BIAS_LOW"=80, "YA_BIAS_OUT"=82, "ZA_BIAS_LOW"=84, "ZA_BIAS_OUT"=86, "Reserved5"=88, "Reserved6"=90, "FILT_CTRL"=92, "Reserved5"=94, "MSC_CTRL"=96, "UP_SCALE"=98, "DEC_RATE"=100, "NULL_CNFG"=102, "GLOB_CMD"=104, "Reserved6"=106, "FIRM_REV"=108, "FIRM_DM"=110, "FIRM_Y"=112, "PROD_ID"=114, "SERIAL_NUM"=116, "USER_SCR1"=118, "USER_SCR2"=120, "USER_SCR3"=122, "FLSHCNT_LOW"=124, "FLSHCNT_HIGH"=126] ("Register")
        w199 = u16 1  # Data
        w194 = T24[] [72, 70, 74] items=["Reserved1"=0, "DIAG_STAT"=2, "X_GYRO_LOW"=4, "X_GYRO_OUT"=6, "Y_GYRO_LOW"=8, "Y_GYRO_OUT"=10, "Z_GYRO_LOW"=12, "Z_GYRO_OUT"=14, "X_ACCL_LOW"=16, "X_ACCL_OUT"=18, "Y_ACCL_LOW"=20, "Y_ACCL_OUT"=22, "Z_ACCL_LOW"=24, "Z_ACCL_OUT"=26, "TEMP_OUT"=28, "TIME_STAMP"=30, "Reseved2"=32, "DATA_CNTR"=34, "X_DELTANG_LOW"=36, "X_DELTANG_OUT"=38, "Y_DELTANG_LOW"=40, "Y_DELTANG_OUT"=42, "Z_DELTANG_LOW"=44, "Z_DELTANG_OUT"=46, "X_DELTVEL_LOW"=48, "X_DELTVEL_OUT"=50, "Y_DELTVEL_LOW"=52, "Y_DELTVEL_OUT"=54, "Z_DELTVEL_LOW"=56, "Z_DELTVEL_OUT"=58, "Reserved3"=60, "Reserved4"=62, "XG_BIAS_LOW"=64, "XG_BIAS_HIGH"=66, "YG_BIAS_LOW"=68, "YG_BIAS_OUT"=70, "ZG_BIAS_LOW"=72, "ZG_BIAS_OUT"=74, "XA_BIAS_LOW"=76, "XA_BIAS_HIGH"=78, "YA_BIAS_LOW"=80, "YA_BIAS_OUT"=82, "ZA_BIAS_LOW"=84, "ZA_BIAS_OUT"=86, "Reserved5"=88, "Reserved6"=90, "FILT_CTRL"=92, "Reserved5"=94, "MSC_CTRL"=96, "UP_SCALE"=98, "DEC_RATE"=100] ("Registers")
        # "Write Calibration"
        # "GLOB_CMD Timing"
        # "Check bias"
        n76 = Unbundle By Name(w186) -> ("ADIS16470DevRef.Status FIFO"=w185:refnum<k33>)
        n77 = Unbundle By Name(w186) -> ("SPIDevRef"=w201:T11)
        n78 = Unbundle By Name(w186) -> ("ADIS16470DevRef.Calibration Complete"=w189:refnum<notifier>)
        n79 = RT FIFO Write(0:w185, 1:T10 {"Calibrated?"=TRUE} ("element")) -> ()  [unwired: 3 in, 4 out]
        n80 = call "ADIS16470 Write Register.vi"("error in (no error)"=w200, "Data"=w199, "Register"=w183, "SPIDevRef in"=w201) -> ("error out"=w198:errorcluster, "SPIDevRef out"=w197:T11)  [unwired: 6 in]
        n81 = flat-sequence {
          tunnel: w198 -> [w205]
          tunnel: [w205] -> w196
          tunnel: w197 -> [w203]
          tunnel: [w203] -> w195
          frame #0 {
            n82 = Wait (ms)(milliseconds to wait=u32 50) -> ()  [unwired: 1 out]
          }
        }
        n83 = call "ADIS16470 Read Multiple Registers.vi"("error in (no error)"=w196, "Registers"=w194, "SPIDevRef"=w195) -> ("error out"=w190:errorcluster, "Values"=w192:u16[])  [unwired: 7 in]
        n84 = To Word Integer(number=w192) -> (16bit integer=→"Offset Bias":i16[])
        n85 = Bundle By Name(cluster=w186, "Yaw"=0.0) -> (w193:T18)
        n86 = Send Notification(notification="", notifier=w189, error in (no error)=w190) -> (error out=w188:errorcluster)  [unwired: 1 out]
      }
      frame "Prepare Run" {
        n87 = call <vilib>:"WPI_DigitalOutputOpen.vi"("error in (no error)"=w208, "DIO Channel"=FPGA_DIOChannel."SPI Port CS3") -> ("error out"=w210:errorcluster, "DigitalOutputDevRef"=w211:T25)  [unwired: 8 in]
        n88 = call <vilib>:"WPI_DigitalOutputClose.vi"("error in (no error)"=w210, "DigitalOutputDevRef"=w211) -> ("error out"=w207:errorcluster)  [unwired: 9 in]
      }
      frame "/***Operation***/" {
      }
      frame "Run" {
        w238 = T24[] [46, 44, 34] items=["Reserved1"=0, "DIAG_STAT"=2, "X_GYRO_LOW"=4, "X_GYRO_OUT"=6, "Y_GYRO_LOW"=8, "Y_GYRO_OUT"=10, "Z_GYRO_LOW"=12, "Z_GYRO_OUT"=14, "X_ACCL_LOW"=16, "X_ACCL_OUT"=18, "Y_ACCL_LOW"=20, "Y_ACCL_OUT"=22, "Z_ACCL_LOW"=24, "Z_ACCL_OUT"=26, "TEMP_OUT"=28, "TIME_STAMP"=30, "Reseved2"=32, "DATA_CNTR"=34, "X_DELTANG_LOW"=36, "X_DELTANG_OUT"=38, "Y_DELTANG_LOW"=40, "Y_DELTANG_OUT"=42, "Z_DELTANG_LOW"=44, "Z_DELTANG_OUT"=46, "X_DELTVEL_LOW"=48, "X_DELTVEL_OUT"=50, "Y_DELTVEL_LOW"=52, "Y_DELTVEL_OUT"=54, "Z_DELTVEL_LOW"=56, "Z_DELTVEL_OUT"=58, "Reserved3"=60, "Reserved4"=62, "XG_BIAS_LOW"=64, "XG_BIAS_HIGH"=66, "YG_BIAS_LOW"=68, "YG_BIAS_OUT"=70, "ZG_BIAS_LOW"=72, "ZG_BIAS_OUT"=74, "XA_BIAS_LOW"=76, "XA_BIAS_HIGH"=78, "YA_BIAS_LOW"=80, "YA_BIAS_OUT"=82, "ZA_BIAS_LOW"=84, "ZA_BIAS_OUT"=86, "Reserved5"=88, "Reserved6"=90, "FILT_CTRL"=92, "Reserved5"=94, "MSC_CTRL"=96, "UP_SCALE"=98, "DEC_RATE"=100] ("Registers")
        # "Sample encoder first since we know the gyro data is good at that timestamp until the next interrupt"
        # "Sample encoders and gyro based on gyro DR interrupt"
        n89 = Unbundle By Name(w222) -> ("SPIDevRef"=w240:T11, "InterruptRef"=w242:T12)
        n90 = Unbundle By Name(w222) -> ("TimeStamp Prev"=w228:dbl)
        n91 = Unbundle By Name(w222) -> ("Encoder Left"=w221:T14, "Encoder Right"=w220:T14)
        n92 = Unbundle By Name(w222) -> ("Yaw"=w229:dbl)
        n93 = call <vilib>:"WPI_InterruptWait.vi"("error in (no error)"=w241, "InterruptRef"=w242) -> ("error out"=w223:errorcluster, "TimeStamp"=w227:dbl)  [unwired: 5 in, 3 out]
        n94 = Subtract(x=w227, y=w228) -> (x-y=w224:dbl)
        n95 = call "ADIS Loop Sample Encoders.vi"("error in (no error)"=w223, "Right Encoder"=w220, "Left Encoder"=w221) -> ("error out"=w217:errorcluster, "cluster"=w219:T26)  [unwired: 7 in]
        n96 = call "ADIS16470 Read Multiple Registers.vi"("error in (no error)"=w217, "Registers"=w238, "SPIDevRef"=w240) -> ("error out"=w239:errorcluster, "Values"=w237:u16[])  [unwired: 7 in]
        n97 = Index Array(array=w237) -> (element #1=w236:u16, element #2=w235:u16, element #3=w216:u16)  [unwired: 3 in]
        n98 = Join Numbers(hi=w236, lo=w235) -> ((hi.lo)=w226:u32)
        n99 = To Long Integer(number=w226) -> (32bit integer=w225:i32)
        n100 = Multiply(x=w225, y=1.005828380585e-08) -> (x*y=w231:dbl)
        n101 = Divide(x=w231, y=w224) -> (x/y=w230:dbl)
        n102 = Add(x=w229, y=w230) -> (x+y=w218:dbl)
        "Waveform Chart" <- w218
        n103 = Bundle By Name(cluster=w222, "Encoder Data"=w219, "Data Counter"=w216, "First Run"=FALSE, "Yaw"=w218, "TimeStamp Prev"=w227, "Time Delta"=w224) -> (w233:T18)
      }
      frame "Process" {
        n104 = Unbundle By Name(w255) -> ("Yaw"=w252:dbl, "TimeStamp Prev"=w253:dbl, "Time Delta"=w250:dbl, "Data Counter"=w251:u16, "Encoder Data"=w246:T26)
        n105 = Bundle By Name(cluster=T9 {"Yaw"=0.0, "Timestamp"=0.0, "Timestamp Delta"=0.0, "Sample Count"=0} ("element"), "Yaw"=w252, "Timestamp"=w253, "Timestamp Delta"=w250, "Sample Count"=w251) -> (w247:T9)
        n106 = call "Sychronous Odometry Processor.vi"("error in (no error)"=w249, "Encoder Data"=w246, "Heading"=w247) -> ("error out"=w248:errorcluster, "Reset?"=w244:bool)  [unwired: 7 in]
        n107 = case shown="True" w244 {
          tunnel: w255 -> [w257 w260]
          tunnel: [w257 w259] -> w245
          frame False {
          }
          frame True {
            n108 = Bundle By Name(cluster=w260, "Yaw"=0.0) -> (w259:T18)
          }
        }
      }
    }
  }
  n109 = call <vilib>:"NetComm_UsageReport_report.vi"("Instance Number"=u8 1, "Resource Type"=NetComm_UsageReport_ResourceType."ADIS16470") -> ()  [unwired: 10 in]
